vi "updateAlly.vi"(8 "error in (no error)":errorcluster, 9 "NavigationTeam":refnum<class "Ally.lvclass">, 10 "Old Ally":refnum<class "Ally.lvclass">, 11 "New Ally from Vision":refnum<class "Ally.lvclass">) -> (0 "error out":errorcluster, 3 "Ally out":refnum<class "Ally.lvclass">)   [LabVIEW 2020, in "Ally.lvclass"]
uses:
  Ally.lvclass
  C:/Users/anton/Desktop/RoboIME/IC/SSL_AI/Team_class/Team.lvclass
  Utilities_class/Utilities.lvclass
  Robot_class/Robot.lvclass
  C:/Users/anton/Desktop/RoboIME/IC/SSL_AI/Object_class/Object.lvclass
  Team_class/Team.lvclass/Team.ctl
  Robot_class/Robot.lvclass/Robot.ctl
  Object_class/Object.lvclass/Object.ctl
  Object_class/Read x.vi
  Object_class/Read y.vi
  Robot_class/Read orientation.vi
  Robot_class/Read est_v_norm.vi
  Robot_class/Read est_v_tang.vi
  Object_class/Read pos_est_x.vi
  Object_class/Read pos_est_y.vi
  Robot_class/Read role.vi
  Object_class/Write x.vi
  Object_class/Write y.vi
  Robot_class/Write orientation.vi
  Robot_class/Write est_v_norm.vi
  Robot_class/Write est_v_tang.vi
  Object_class/Write pos_est_x.vi
  Object_class/Write pos_est_y.vi
  Robot_class/Write role.vi
  Robot_class/Read id.vi
  Team_class/Read RobotRef.vi
  Team_class/Write RobotRef.vi
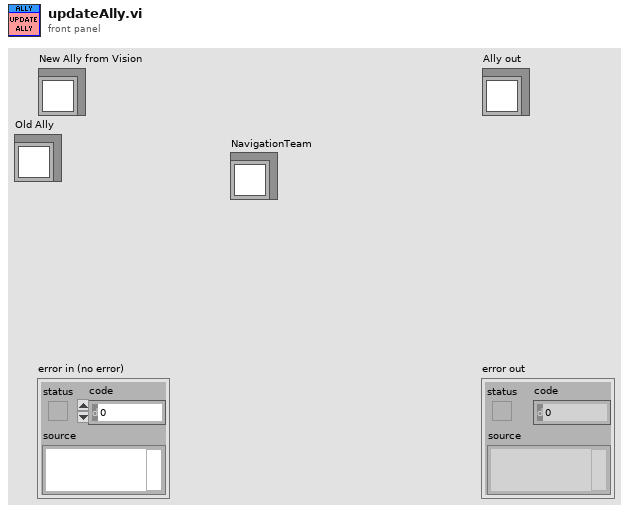
[diagram p1: front panel]
types:
  T1 = typedef "roles.ctl" = enum16{"SimpleBallPlacement", "BallPlacementAllyPasser", "BallPlacementAllyReceiver", "BallPlacementEnemy", "5Robots5th", "PassBestReceiver", "5Robots4th", "5Robots3rd", "5Robots2nd", "5Robots1st", "PassBestRobot", "WaitPass", "ABCThirdKicker", "ABCFirstKicker", "ABCSecondKicker", "Tabler", "TableFinalizer", "PrepareRollToPassRoller", "PrepareRollToPassReceiver", "SimplePassRoll", "SimplePassRollReceiver", "PenaltyDefense", "PreparePassReceiver 2", "PreparePassReceiver 1", "PassObserver", "Timeout", "Goto", "ZigZag", "None", "BallOutOfField", "DefenderArea", "Duelist", "AttackerStop", "FollowAttacker", "KeeperRole", "KickPenalty", "AttackerAimGoal", "AttackerBlock", "Marker", "Halt", "Shoot", "PassKicker", "PassReceiver", "TestRole", "PenaltyAttacker"}
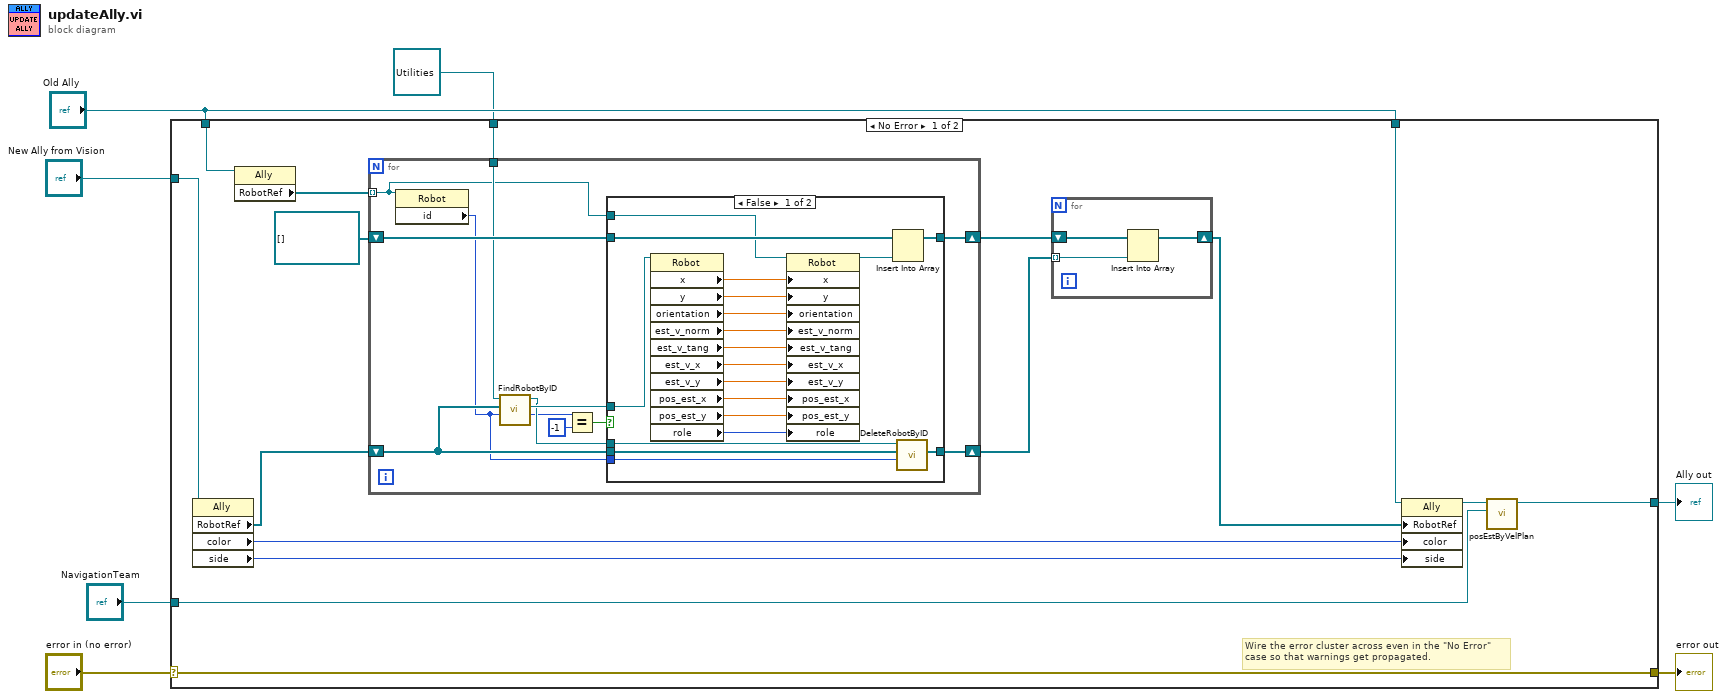
[diagram p0: block diagram]
diagram:
  n1 = case shown="No Error" "error in (no error)" {
    selector: "error in (no error)" -> [w23 w61]
    tunnel: [w23 w61] -> w6
    tunnel: [w8 w60] -> w4
    tunnel: "New Ally from Vision" -> [w22 w60]
    tunnel: "Old Ally" -> [w21 _]
    tunnel: "Old Ally" -> [w18 _]
    tunnel: refnum<class "Utilities.lvclass"> refnum ("Utilities in") -> [w14 _]
    tunnel: "NavigationTeam" -> [w9 _]
    frame No Error {
      # "Wire the error cluster across even in the \"No Error\"\ncase so that warnings get propagated."
      n2 = property class="Ally"(reference=w22) -> ("RobotRef"=w17:refnum<class "Robot.lvclass">[], "color"=w20:enum16{"Azul", "Amarelo"}, "side"=w19:enum16{"Esquerdo", "Direito"})  [unwired: 1 in, 2 out]
      n3 = property class="Ally"(reference=w18) -> ("RobotRef"=w16:refnum<class "Robot.lvclass">[])  [unwired: 1 in, 2 out]
      n4 = for {
        tunnel: w16 -> [w27] mode=indexing
        shift-right: [w37] -> w13
        shift-left: refnum<class "Robot.lvclass">[] [] -> [w36]
        tunnel: w14 -> [w35]
        shift-right: [w32] -> w12
        shift-left: w17 -> [w34]
        n5 = property class="Robot"(reference=w27) -> ("id"=w33:i32)  [unwired: 1 in, 2 out]
        n6 = call "FindRobotByID.vi"("id"=w33, "RobotRef"=w34, "Utilities in"=w35) -> ("index"=w29:i32, "Robot"=w38:refnum<class "Robot.lvclass">, "Utilities out"=w31:refnum<class "Utilities.lvclass">)  [unwired: 5 in, 1 out]
        n7 = Equal?(x=w29, y=-1) -> (x = y?=w30:bool)
        n8 = case shown="False" w30 {
          tunnel: w38 -> [w49 _]
          tunnel: [w57 w59] -> w37
          tunnel: w36 -> [w56 w59]
          tunnel: w34 -> [w55 w58]
          tunnel: w33 -> [w54 _]
          tunnel: [w53 w58] -> w32
          tunnel: w31 -> [w52 _]
          tunnel: w27 -> [w51 _]
          frame False {
            n9 = property class="Robot"(reference=w49) -> ("x"=w48:dbl, "y"=w47:dbl, "orientation"=w46:dbl, "est_v_norm"=w45:dbl, "est_v_tang"=w44:dbl, "est_v_x"=w43:dbl, "est_v_y"=w42:dbl, "pos_est_x"=w41:dbl, "pos_est_y"=w40:dbl, "role"=w39:T1)  [unwired: 1 in, 2 out]
            n10 = property class="Robot"(reference=w51, "x"=w48, "y"=w47, "orientation"=w46, "est_v_norm"=w45, "est_v_tang"=w44, "est_v_x"=w43, "est_v_y"=w42, "pos_est_x"=w41, "pos_est_y"=w40, "role"=w39) -> (reference out=w50:refnum<class "Robot.lvclass">)  [unwired: 1 in, 1 out]
            n11 = Insert Into Array(array=w56, new element=w50) -> (w57:refnum<class "Robot.lvclass">[])  [unwired: 1 in]
            n12 = call "DeleteRobotByID.vi"("id"=w54, "RobotRef"=w55, "Utilities in"=w52) -> ("RobotRef out"=w53:refnum<class "Robot.lvclass">[])  [unwired: 6 in, 2 out]
          }
          frame True {
          }
        }
      }
      n13 = for {
        shift-right: [w24] -> w11
        shift-left: w13 -> [w26]
        tunnel: w12 -> [w25] mode=indexing
        n14 = Insert Into Array(array=w26, new element=w25) -> (w24:refnum<class "Robot.lvclass">[])  [unwired: 1 in]
      }
      n15 = property class="Ally"(reference=w21, "RobotRef"=w11, "color"=w20, "side"=w19) -> (reference out=w10:refnum<class "Ally.lvclass">)  [unwired: 1 in, 1 out]
      n16 = call "posEstByVelPlan.vi"("NavigationTeam"=w9, "Ally in"=w10) -> ("Ally out"=w8:refnum<class "Ally.lvclass">)  [unwired: 8 in, 1 out]
    }
    frame Error {
    }
  }
  "error out" <- w6
  "Ally out" <- w4
